vi "Shooter Calculations.vi"() -> ()   [LabVIEW 2011]
uses:
  Globals/Load Cell Multiplier.vi
  Globals/Calculated Shooter Speed.vi
  Globals/Image Height.vi
  Globals/Alignment Error.vi
panel:
  in  "Center of Mass X":dbl=298.96
  out "Load Cell Max Value":dbl=0.554001806
  out "Sensor Plot":dbl(graph)=0.5385810950000001
  out "Load Cell RT Value":dbl=0.5385810950000001
  out "axis 3 (throttle)":dbl=0.11023622047244094
  out "Aiming Error":dbl=-21.04000000000002
  out "Raw String from UDP":string="!195,298.96,173.18,132.00,92.00,461.31,366.92,129.00,105.00,143.32,371.39,129.00,97.00,#END"
  out "Center of Mass X 2":dbl(graph)=298.96
  in  "Axis 3":dbl=0.11023622047244094
  out "Load Cell Multiplier":dbl=1.0
  out "Driver Multiplier":dbl=0.9944881889763779
  in  "Correction":dbl
  in  "Manual Multiplier":dbl=1.0
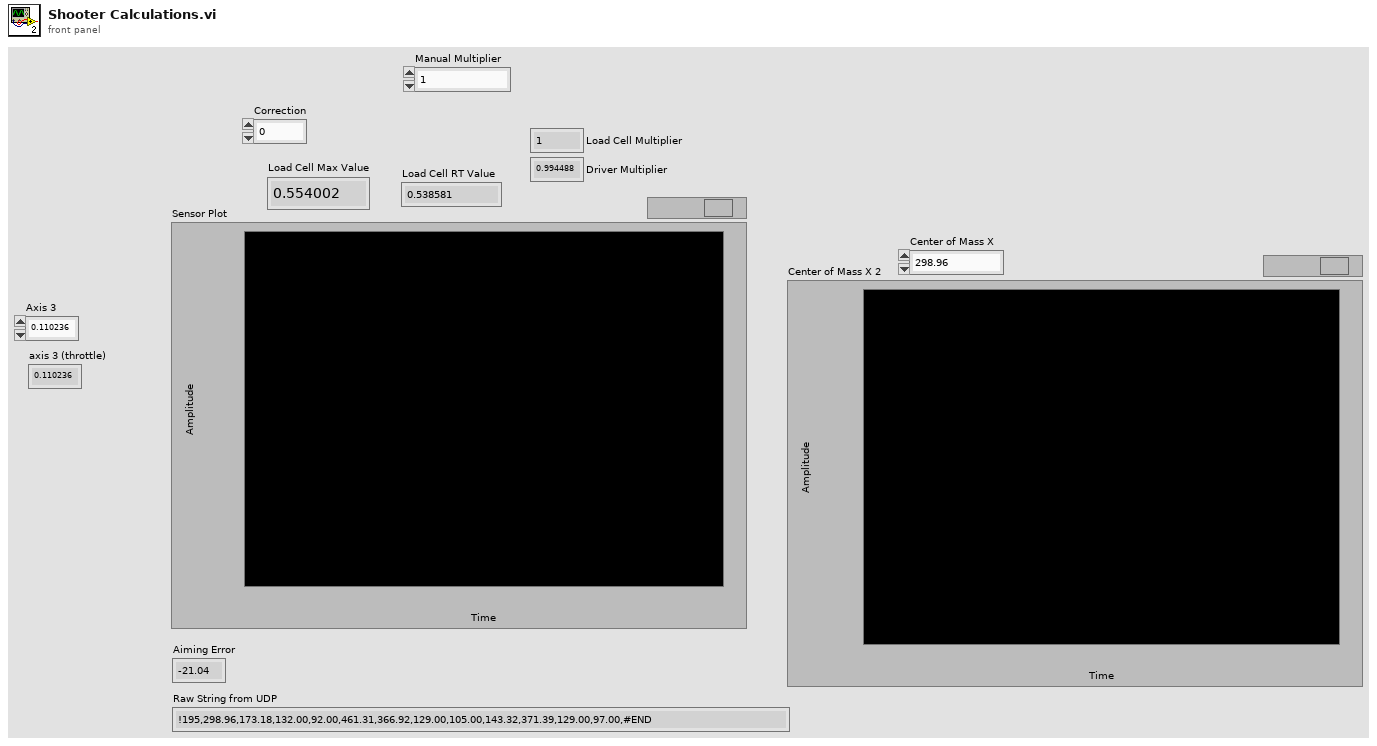
[diagram p1: front panel]
types:
  T1 = typedef "WPI_AnalogChannelDevRef.ctl" = cluster{"DevStatus":errorcluster, "Analog Module":T2, "Analog Channel":T3}
  T2 = typedef "FPGA_TypedefAnalogModule.ctl" = enum16{"Analog Module 1", "Analog Module 2"}
  T3 = typedef "FPGA_AIChannel.ctl" = enum8{"AI 1", "AI 2", "AI 3", "AI 4", "AI 5", "AI 6", "AI 7", "AI 8", "Invalid"}
  T4 = typedef "WPI_JoystickDevRef.ctl" = cluster{"Device":T5}
  T5 = typedef "WPI_JoystickDeviceEnum.ctl" = enum16{"USB 1", "USB 2", "USB 3", "USB 4", "Kinect 1", "Kinect 2"}
  T6 = typedef "WPI_JoystickButtonState.ctl" = cluster{"Button 1":bool, "Button 2":bool, "Button 3":bool, "Button 4":bool, "Button 5":bool, "Button 6":bool, "Button 7":bool, "Button 8":bool, "Button 9":bool, "Button 10":bool, "Button 11":bool, "Button 12":bool}
  T7 = typedef "WPI_GyroDevRef.ctl" = cluster{"DevStatus":errorcluster, "Analog Module":T2, "Analog Channel":T3, "Offset":dbl, "Gain (VoltsPerDegree/Second)":dbl}
  T8 = cluster{"axis 1 (x)":dbl, "axis 2 (y)":dbl, "axis 3 (throttle)":dbl, "axis 4":dbl, "axis 5":dbl, "axis 6":dbl}
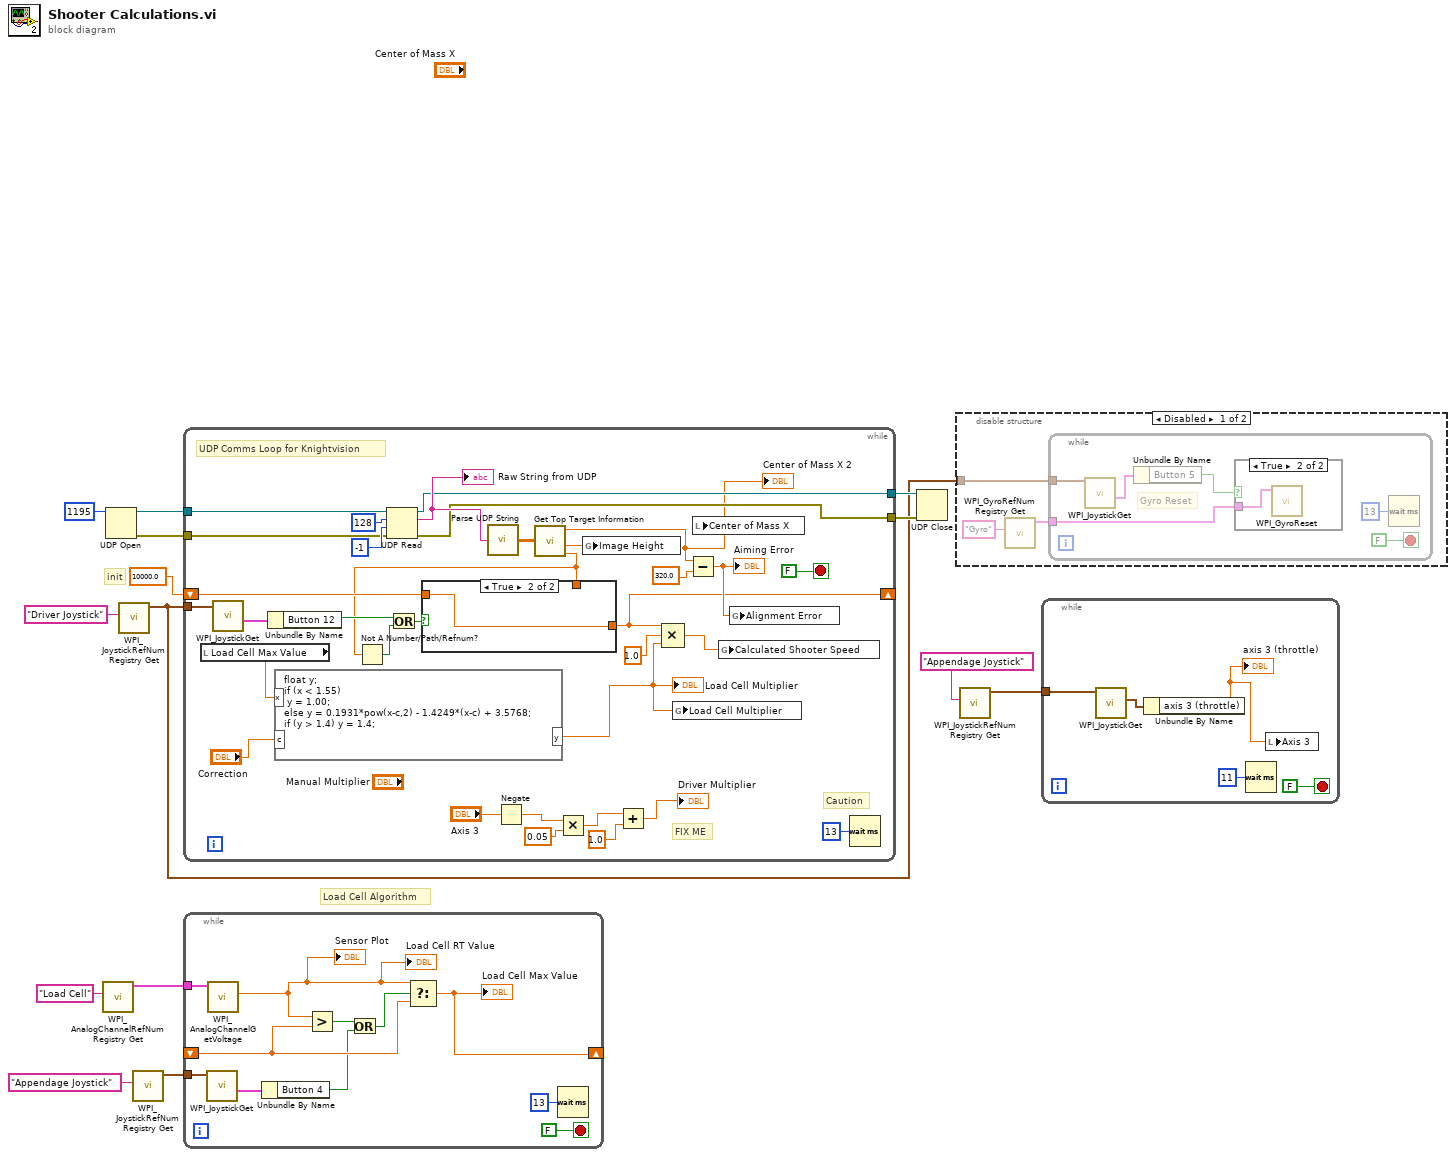
[diagram p0: block diagram]
diagram:
  # "Load Cell Algorithm"
  # "init"
  n1 = call <vilib>:"WPI_AnalogChannelRefNum Registry Get.vi"("refnum name"="Load Cell") -> ("AIDeviceRef"=w4:T1)  [unwired: 9 in, 1 out]
  n2 = UDP Open(11:u16 1195 ("port")) -> (port=w13:refnum<k16>, 0:w12:errorcluster)  [unwired: 4 in, 1 out]
  n3 = call <vilib>:"WPI_JoystickRefNum Registry Get.vi"("refnum name"="Driver Joystick") -> ("JoystickDevRef"=w3:T4)  [unwired: 9 in, 1 out]
  n4 = call <vilib>:"WPI_JoystickRefNum Registry Get.vi"("refnum name"="Appendage Joystick") -> ("JoystickDevRef"=w1:T4)  [unwired: 9 in, 1 out]
  n5 = while {
    tunnel: w13 -> [w41]
    tunnel: w12 -> [w40]
    tunnel: [w39] -> w11
    tunnel: [w38] -> w10
    shift-right: [w26] -> _
    shift-left: 10000.0 ("Calculated Shooter Speed") -> [w36]
    tunnel: w3 -> [w34]
    stop <- FALSE stop-if-true
    # "Caution"
    # "FIX ME"
    # "UDP Comms Loop for Knightvision"
    n6 = local read "Load Cell Max Value"() -> (w25:dbl)
    n7 = call <vilib>:"WPI_JoystickGet.vi"("JoystickDevRef"=w34) -> ("Buttons"=w35:T6)  [unwired: 4 in, 2 out]
    n8 = Unbundle By Name(w35) -> ("Button 12"=w31:bool)
    n9 = formula code="float y;\nif (x < 1.55)\n y = 1.00;\nelse y = 0.1931*pow(x-c,2) - 1.4249*(x-c) + 3.5768;\nif (y > 1.4) y = 1.4;"("x"=w25, "c"="Correction") -> ("y"=w16:dbl)
    "Load Cell Multiplier" <- w16
    n10 = UDP Read(connection ID=w41, max size (548)=128, timeout ms (25000)=-1, 8:w40) -> (data out=w46:string, error out=w38:errorcluster, 3:w39:refnum<k16>)  [unwired: 2 out]
    "Raw String from UDP" <- w46
    n11 = call "Parse UDP String.vi"("UDP Packet In"=w46) -> ("Array"=w43:dbl[][])
    n12 = Negate(x="Axis 3") -> (-x=w21:dbl)
    n13 = call "Get Top Target Information.vi"("Vision Info Array"=w43) -> ("Center of Mass X"=w37:dbl, "Bounding Box Height"=w32:dbl, "Calculated Shooter Speed"=w29:dbl)  [unwired: 1 out]
    "Center of Mass X 2" <- w37
    n14 = Not A Number/Path/Refnum?(number/path/refnum=w29) -> (NaN/Path/Refnum?=w28:bool)
    n15 = Or(x=w31, y=w28) -> (x .or. y?=w30:bool)
    n16 = case shown="True" w30 {
      tunnel: w29 -> [w48 _]
      tunnel: [w48 w49] -> w26
      tunnel: w36 -> [_ w49]
      frame False {
      }
      frame True {
      }
    }
    n17 = Multiply(x=w21, y=0.05) -> (x*y=w22:dbl)
    n18 = global write "Image Height.vi" "Image Height"(w32) -> ()
    n19 = Add(x=w22, y=1.0) -> (x+y=→"Driver Multiplier":dbl)
    n20 = Compound Arithmetic op=MULTIPLY(w26, 1.0 ("value"), w16) -> (w27:dbl)
    n21 = global write "Load Cell Multiplier.vi" "Load Cell Multiplier"(w16) -> ()
    n22 = Subtract(x=w37, y=320.0) -> (x-y=w33:dbl)
    "Aiming Error" <- w33
    n23 = local write "Center of Mass X"(w37) -> ()
    n24 = global write "Calculated Shooter Speed.vi" "Calculated Shooter Speed"(w27) -> ()
    n25 = global write "Alignment Error.vi" "Alignment Error"(w33) -> ()
    n26 = Wait (ms)(milliseconds to wait=u32 13) -> ()  [unwired: 1 out]
  }
  n27 = while {
    tunnel: w4 -> [w60]
    shift-right: [w51] -> _
    shift-left: _ -> [w57]
    tunnel: w1 -> [w55]
    stop <- FALSE stop-if-true
    n28 = call <vilib>:"WPI_JoystickGet.vi"("JoystickDevRef"=w55) -> ("Buttons"=w54:T6)  [unwired: 4 in, 2 out]
    n29 = call <vilib>:"WPI_AnalogChannelGetVoltage.vi"("AIDeviceRef"=w60) -> ("Voltage"=w50:dbl)  [unwired: 8 in, 2 out]
    "Sensor Plot" <- w50
    "Load Cell RT Value" <- w50
    n30 = Unbundle By Name(w54) -> ("Button 4"=w53:bool)
    n31 = Greater?(x=w50, y=w57) -> (0:w56:bool)
    n32 = Or(x=w56, y=w53) -> (x .or. y?=w52:bool)
    n33 = Select(t=w50, s=w52, f=w57) -> (s? t:f=w51:dbl)
    "Load Cell Max Value" <- w51
    n34 = Wait (ms)(milliseconds to wait=u32 13) -> ()  [unwired: 1 out]
  }
  n35 = UDP Close(connection ID=w11, 8:w10) -> ()  [unwired: 2 out]
  n36 = disable-structure shown="Disabled" {
    disable-tunnel: w3 -> [w61 _]
    frame Disabled {
      n37 = call <vilib>:"WPI_GyroRefNum Registry Get.vi"("refnum name"="Gyro") -> ("GyroDevRef"=w62:T7)  [unwired: 9 in, 1 out]
      n38 = while {
        tunnel: w61 -> [w66]
        tunnel: w62 -> [w64]
        stop <- FALSE stop-if-true
        # "Gyro Reset"
        n39 = call <vilib>:"WPI_JoystickGet.vi"("JoystickDevRef"=w66) -> ("Buttons"=w67:T6)  [unwired: 4 in, 2 out]
        n40 = Unbundle By Name(w67) -> ("Button 5"=w65:bool)
        n41 = case shown="True" w65 {
          tunnel: w64 -> [_ w70]
          frame False {
          }
          frame True {
            n42 = call <vilib>:"WPI_GyroReset.vi"("GyroDevRef"=w70) -> ()  [unwired: 9 in, 2 out]
          }
        }
        n43 = Wait (ms)(milliseconds to wait=u32 13) -> ()  [unwired: 1 out]
      }
    }
    frame Enabled {
    }
  }
  n44 = call <vilib>:"WPI_JoystickRefNum Registry Get.vi"("refnum name"="Appendage Joystick") -> ("JoystickDevRef"=w7:T4)  [unwired: 9 in, 1 out]
  n45 = while {
    tunnel: w7 -> [w74]
    stop <- FALSE stop-if-true
    n46 = call <vilib>:"WPI_JoystickGet.vi"("JoystickDevRef"=w74) -> ("Axes"=w75:T8)  [unwired: 4 in, 2 out]
    n47 = Unbundle By Name(w75) -> ("axis 3 (throttle)"=w71:dbl)
    "axis 3 (throttle)" <- w71
    n48 = Wait (ms)(milliseconds to wait=u32 11) -> ()  [unwired: 1 out]
    n49 = local write "Axis 3"(w71) -> ()
  }
